vi "art联动采集V4.3.vi"() -> ()   [LabVIEW 2016]
uses:
  <vilib>/Instr/_visa.llb/VISA Configure Serial Port (Instr).vi
  <vilib>/Utility/file.llb/Write Delimited Spreadsheet (DBL).vi
panel:
  in  "定位模式":bool
  in  "X终点":dbl
  in  "Y终点":dbl
  in  "高级设置":bool
  in  "Y轴回零速度":dbl=15000.0
  in  "X轴回零速度":dbl=15000.0
  in  "细分设置":dbl=8.0
  in  "等待时间":u32=40
  in  "文件保存":path=path "C:/Users/H301/Desktop/art采集实验数据" caption="保存路径"
  out "行用时（s）":dbl
  out "time（行）":u32
  out "hDevice out":i32=253955776
  out "error out":errorcluster caption="错误输出"
  in  "退出扫描(Esc)":bool
  in  "N_Length":i32=16384
  out "M_Length":i32
  out "hDevice":i32=241832032
  out "pulDDR2Length":u32=256
  out "总用时（s）":dbl
  out "毫秒计时值":u32=3586537
  out "数组":dbl[][](array[numeric])=[[58819.77200735986, 88200.32943600747]]
  out "强度图":dbl[][](graph)=[[58819.77200735986, 88200.32943600747]]
  out "judge":dbl
  out "Xloop":dbl
  out "幅频谱":dbl[](graph)
  out "时域谱":dbl[](graph)
  out "错误输出":errorcluster
  in  "启动":bool
  in  "开始扫描":bool
  in  "X归零":bool
  in  "Y归零":bool
  in  "Y起点":dbl
  in  "Y轴速度":dbl=9000.0
  in  "X轴速度":dbl=9000.0
  out "电机状态":bool
  in  "电机端口":refnum<visa-resource-name>="COM6"
  out "Yloop":dbl=1.0
  out "X扫描范围":dbl=150.0
  out "Y扫描范围":dbl=75.0
  out "Y序":i32
  in  "X起点":dbl
  out "Y(mm)":dbl
  out "x+y 2":dbl=3.0
  in  "Y步进":dbl=1.0
  in  "精度":dbl=0.001
  in  "电机急停":bool
  out "X（mm）":dbl
  out "x+y":dbl=1.0
  in  "X步进":dbl=1.0
  # "实时坐标"
  # "时域谱"
  # "频域谱"
  # "扫描参数"
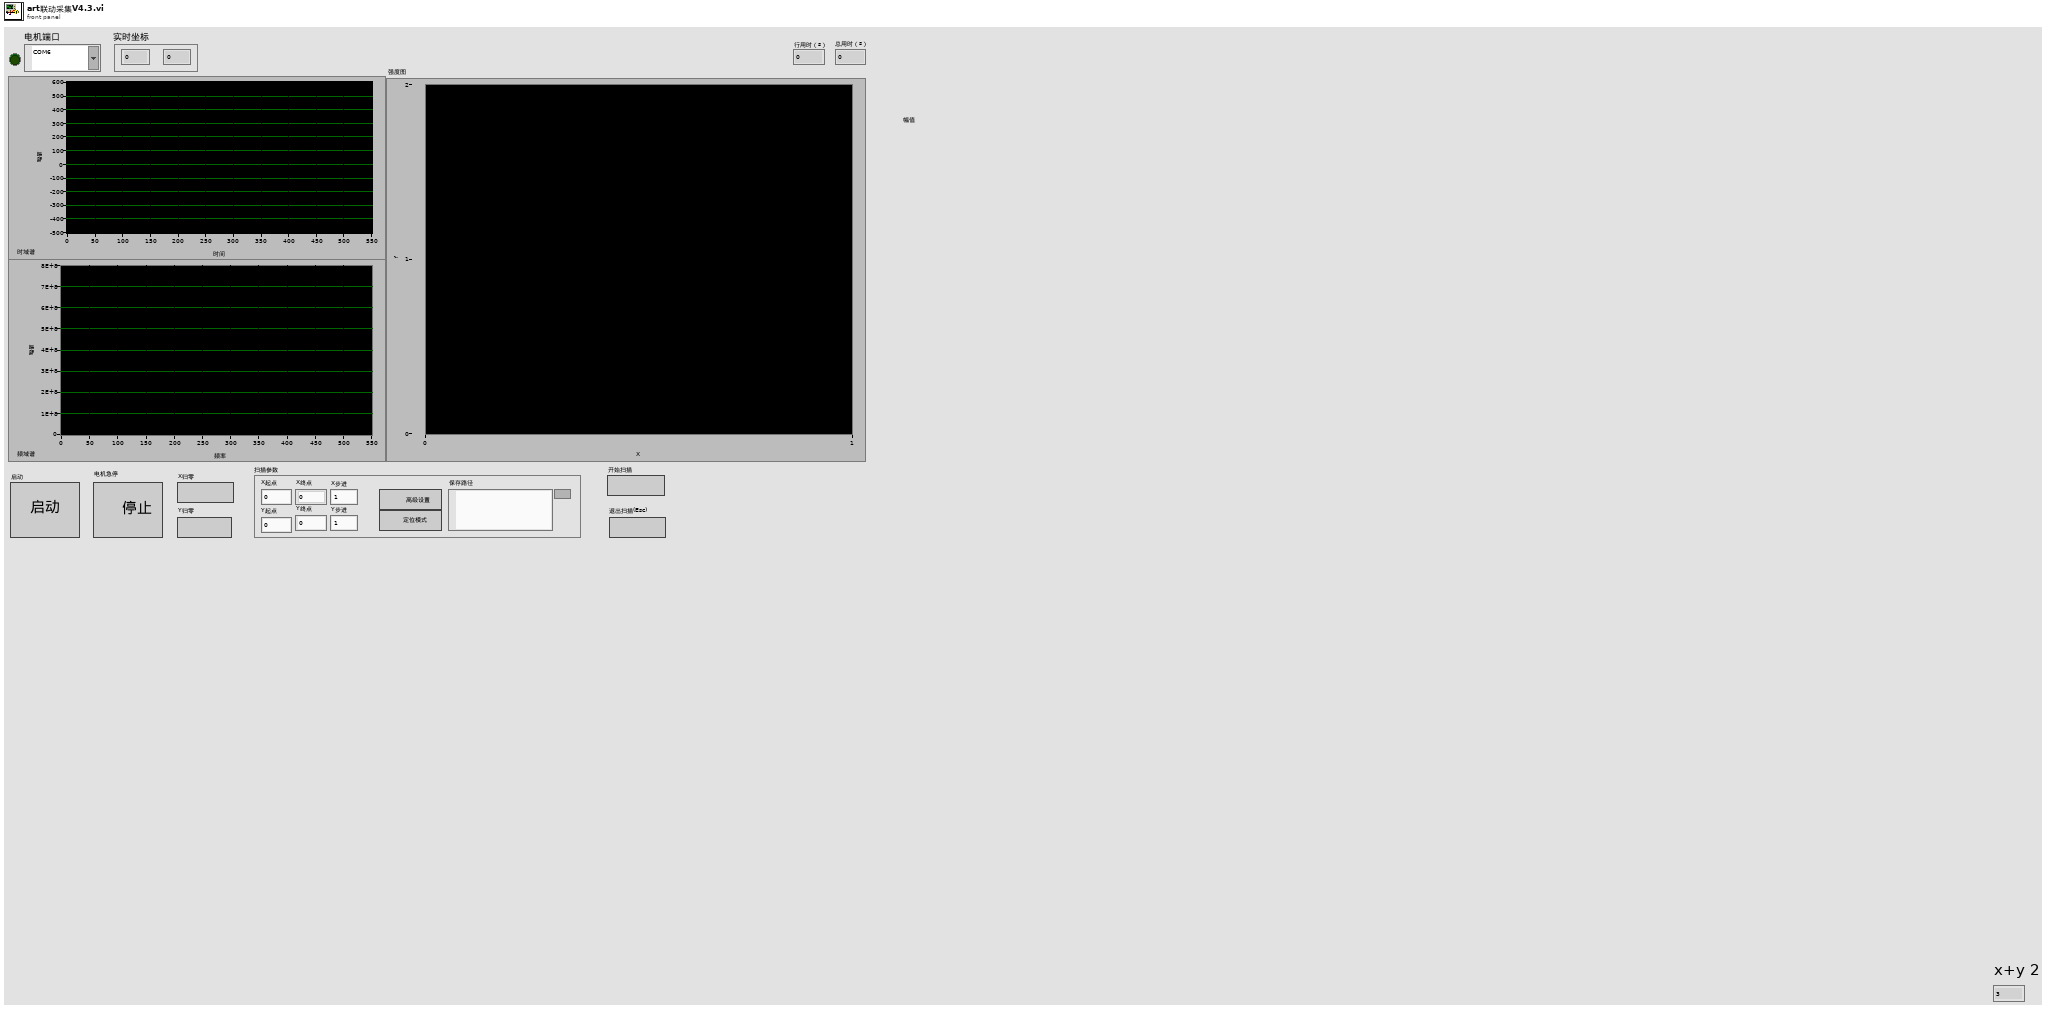
[diagram p1: front panel]
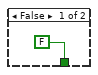
[diagram p2: hidden frame]
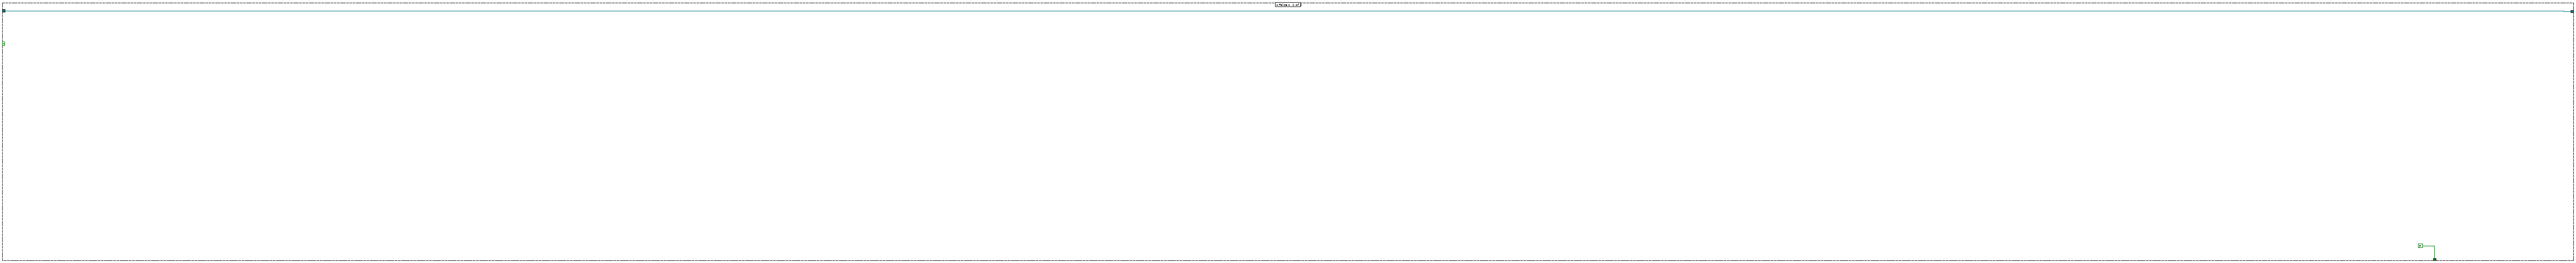
[diagram p3: hidden frame]
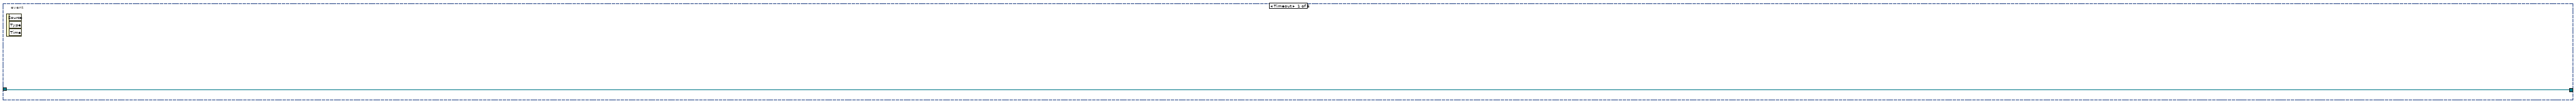
[diagram p4: hidden frame]
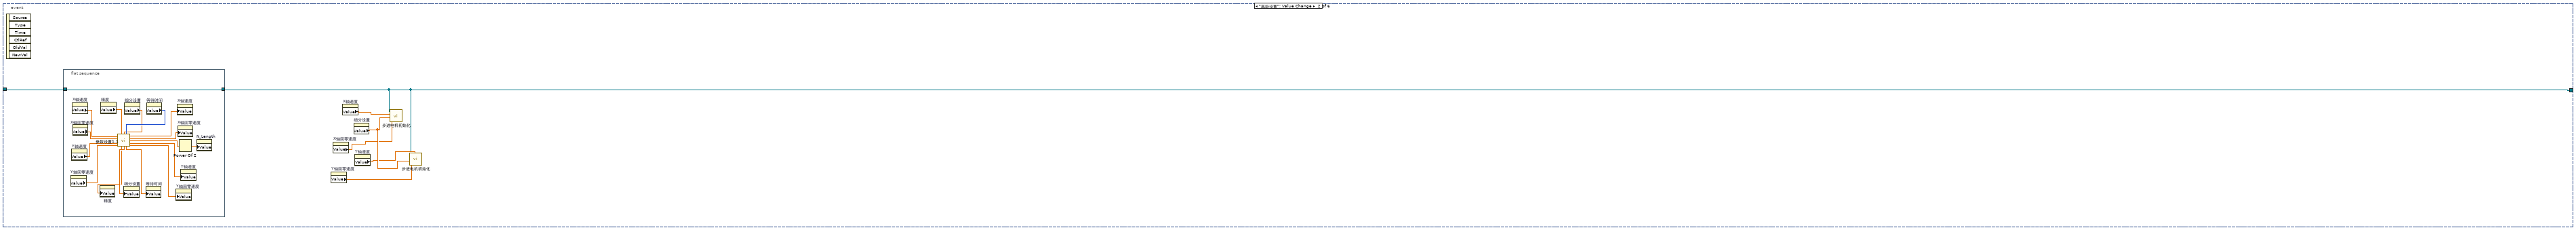
[diagram p5: hidden frame]
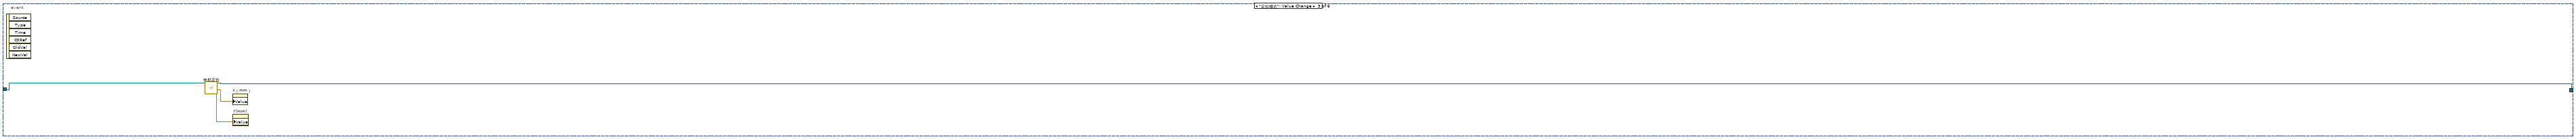
[diagram p6: hidden frame]
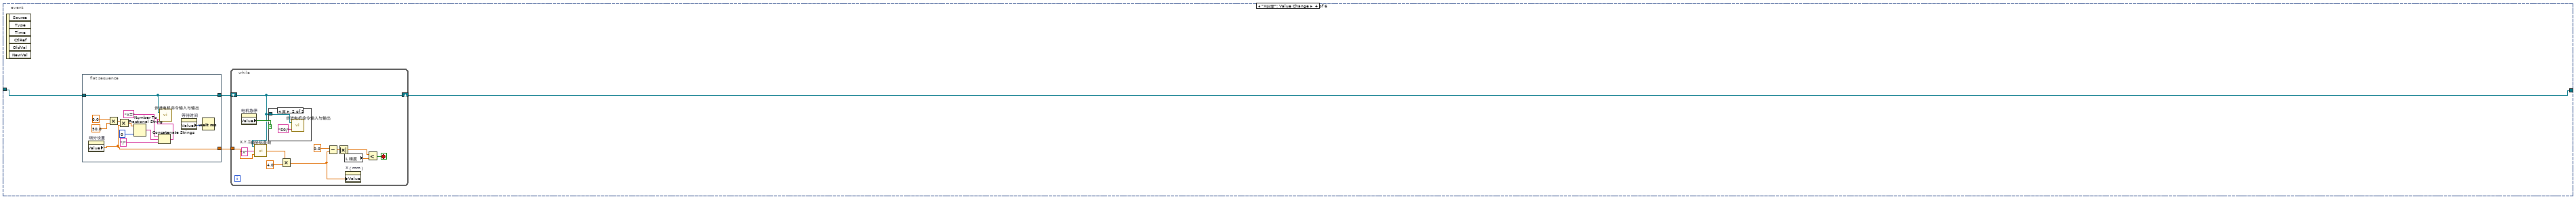
[diagram p7: hidden frame]
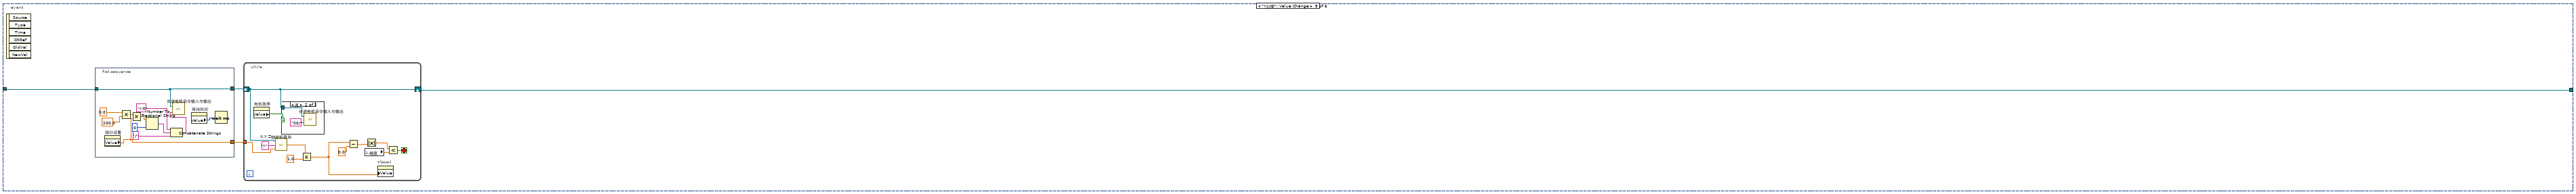
[diagram p9: hidden frame]
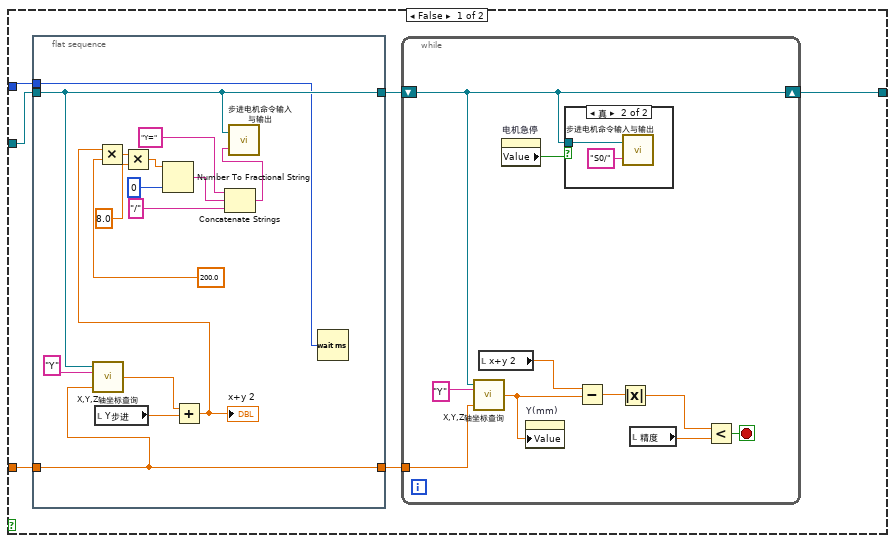
[diagram p14: hidden frame]
diagram:
  n1 = while {
    stop <- w3 stop-if-true
    n2 = case shown="真" "启动" {
      tunnel: [FALSE ("ESC") w11] -> w3
      frame False {
      }
      frame True {
        w25 = 0  # OutClockSource
        w26 = 0  # bClockSourceDir
        w28 = 10000000  # Frequency
        w29 = 0  # ClockSource
        w30 = 0  # TrigLevelVolt
        w18 = 1
        w31 = 0  # TriggerDir
        w32 = 0  # TriggerSource
        w33 = 0  # ATRTriggerChannel
        w34 = 0  # TriggerMode
        w19 = 0  # M_Length
        w35 = 1  # CouplingType
        w36 = 0  # DeviceLgcID
        w46 = u16 0 items=["无", "XON/XOFF", "RTS/CTS", "XON/XOFF & RTS/CTS", "DTR/DSR", "XON/XOFF & DTR/DSR"] ("flow control (0:none)")
        w47 = u16 10 items=["1.0"=10, "1.5"=15, "2.0"=20] ("stop bits (10: 1 bit)")
        # "3"
        # "2"
        # "1"
        n3 = call-poly "VISA Configure Serial Port"("VISA resource name"="电机端口", "baud rate (9600)"=u32 9600, "data bits (8)"=u16 8, "parity (0:none)"=enum16{"None", "Odd", "Even", "Mark", "Space"}."None", "stop bits (10: 1 bit)"=w47, "flow control (0:none)"=w46) -> ("VISA resource name out"=w38:refnum<visa-resource-name>, "error out"=→"error out":errorcluster)  [unwired: 1 in, 7 out]
        n4 = Build Array "InputRange"(w18, w18, w18, w18) -> (w17:i32[])
        n5 = dll-call lib="PTH2aabs CUsersH301Desktopart闭环扫描程序采集卡控制INFamd64PCI8502_32.dll" fn="PCI8502_CreateDevice" label="CreateDevice"("DeviceLgcID"=w36) -> (w23:i32)  [unwired: 4 in, 2 out]
        n6 = property on="细分设置" class="DigNum (严格)"() -> ("Value"=w10:dbl)  [unwired: 2 in, 2 out]
        n7 = Build Array (concatenate) "InitDeviceAD"(w28, w17, w35, w19, "N_Length", w34, w33, w32, w31, w30, w29, w26, w25) -> (w27:i32[])
        n8 = call "步进电机初始化.vi"("回零速度"="X轴回零速度", "细分设置"=w10, "X轴速度"="X轴速度", "串口通信端口"=w38) -> ()  [unwired: 2 in, 1 out]
        n9 = dll-call lib="PTH2aabs CUsersH301Desktopart闭环扫描程序采集卡控制INFamd64PCI8502_32.dll" fn="PCI8502_GetDDR2Length" label="GetDDR2Length"("hDevice"=w23, "pulDDR2Length"=u32 0) -> ("hDevice"=w22:i32, "pulDDR2Length"=→"pulDDR2Length":u32)  [unwired: 4 in, 2 out]
        n10 = call "步进电机初始化.vi"("Y轴速度"="Y轴速度", "回零速度"="Y轴回零速度", "细分设置"=w10, "串口通信端口"=w38) -> ()  [unwired: 2 in, 1 out]
        n11 = call "步进电机命令输入与输出.vi"("输入字符串"="?R/", "串口通信端口"=w38) -> ("返回字符串"=w43:string)
        n12 = dll-call lib="PTH2aabs CUsersH301Desktopart闭环扫描程序采集卡控制INFamd64PCI8502_32.dll" fn="PCI8502_InitDeviceAD" label="InitDeviceAD"("hDevice"=w22, "pADPara"=w27) -> ("hDevice"=→"hDevice":i32)  [unwired: 5 in, 2 out]
        n13 = String Subset(string=w43, offset (0)=0 ("偏移量(0)"), length (rest)=2 ("长度（剩余）")) -> (substring=w40:string)
        n14 = Equal?(x=w40, y="OK") -> (x = y?=w37:bool)
        "电机状态" <- w37
        n15 = case shown="真" w37 {
          tunnel: w38 -> [w53 w56]
          tunnel: [w53 w54] -> w12
          tunnel: [FALSE ("ESC") w55] -> w11
          frame False {
          }
          frame True {
            n16 = while {
              tunnel: ["退出扫描(Esc)"] -> w55
              shift-right: [w57] -> w54
              shift-left: w56 -> [w62]
              stop <- "退出扫描(Esc)" stop-if-true
              n17 = property on="高级设置" class="Bool"("Visible"=TRUE ("可见")) -> ()  [unwired: 2 in, 2 out]
              n18 = property on="定位模式" class="Bool"("Visible"=TRUE ("可见")) -> ()  [unwired: 2 in, 2 out]
              n19 = event shown="[5] \"开始扫描\": 值改变" {
                selector: _ -> [_ _ _ _ _ _]
                dyn-events: _ -> [_ _ _ _ _ _]
                timeout: 1 -> [_ _ _ _ _ _]
                tunnel: w62 -> [w63 w70 w91 w95 w125 w176]
                tunnel: [w63 w64 w90 w93 w123 w170] -> w57
                event Timeout {
                  n20 = event-data() -> ()  [unwired: 1 in, 3 out]
                }
                event "高级设置": Value Change {
                  n21 = event-data() -> ()  [unwired: 1 in, 6 out]
                  n22 = flat-sequence {
                    tunnel: w70 -> [w73]
                    tunnel: [w73] -> w64
                    frame #0 {
                      n23 = property on="Y轴回零速度" class="DigNum (严格)"() -> ("Value"=w77:dbl)  [unwired: 2 in, 2 out]
                      n24 = property on="Y轴速度" class="DigNum (严格)"() -> ("Value"=w76:dbl)  [unwired: 2 in, 2 out]
                      n25 = property on="X轴速度" class="DigNum (严格)"() -> ("Value"=w74:dbl)  [unwired: 2 in, 2 out]
                      n26 = property on="X轴回零速度" class="DigNum (严格)"() -> ("Value"=w75:dbl)  [unwired: 2 in, 2 out]
                      n27 = property on="精度" class="DigNum (严格)"() -> ("Value"=w81:dbl)  [unwired: 2 in, 2 out]
                      n28 = property on="细分设置" class="DigNum (严格)"() -> ("Value"=w82:dbl)  [unwired: 2 in, 2 out]
                      n29 = property on="等待时间" class="DigNum (严格)"() -> ("Value"=w83:u32)  [unwired: 2 in, 2 out]
                      n30 = call "参数设置1.1.vi"("X轴速度"=w74, "精度"=w81, "细分设置"=w82, "等待时间"=w83, "X轴回零速度"=w75, "Y轴速度"=w76, "Y轴回零速度"=w77) -> ("X轴速度"=w84:dbl, "X轴回零速度"=w85:dbl, "采样阶"=w71:dbl, "Y轴速度"=w86:dbl, "精度"=w78:dbl, "细分设置"=w79:dbl, "等待时间"=w80:dbl, "Y轴回零速度"=w87:dbl)  [unwired: 1 in]
                      n31 = property on="精度" class="DigNum (严格)"("Value"=w78) -> ()  [unwired: 2 in, 2 out]
                      n32 = property on="细分设置" class="DigNum (严格)"("Value"=w79) -> ()  [unwired: 2 in, 2 out]
                      n33 = property on="等待时间" class="DigNum (严格)"("Value"=w80) -> ()  [unwired: 2 in, 2 out]
                      n34 = property on="Y轴回零速度" class="DigNum (严格)"("Value"=w87) -> ()  [unwired: 2 in, 2 out]
                      n35 = property on="X轴速度" class="DigNum (严格)"("Value"=w84) -> ()  [unwired: 2 in, 2 out]
                      n36 = property on="X轴回零速度" class="DigNum (严格)"("Value"=w85) -> ()  [unwired: 2 in, 2 out]
                      n37 = Power Of 2(x=w71) -> (2^x=w72:dbl)
                      n38 = property on="Y轴速度" class="DigNum (严格)"("Value"=w86) -> ()  [unwired: 2 in, 2 out]
                      n39 = property on="N_Length" class="DigNum (严格)"("Value"=w72) -> ()  [unwired: 2 in, 2 out]
                    }
                  }
                  n40 = property on="Y轴回零速度" class="DigNum (严格)"() -> ("Value"=w66:dbl)  [unwired: 2 in, 2 out]
                  n41 = property on="X轴回零速度" class="DigNum (严格)"() -> ("Value"=w67:dbl)  [unwired: 2 in, 2 out]
                  n42 = property on="X轴速度" class="DigNum (严格)"() -> ("Value"=w68:dbl)  [unwired: 2 in, 2 out]
                  n43 = property on="细分设置" class="DigNum (严格)"() -> ("Value"=w69:dbl)  [unwired: 2 in, 2 out]
                  n44 = property on="Y轴速度" class="DigNum (严格)"() -> ("Value"=w65:dbl)  [unwired: 2 in, 2 out]
                  n45 = call "步进电机初始化.vi"("回零速度"=w67, "细分设置"=w69, "X轴速度"=w68, "串口通信端口"=w64) -> ()  [unwired: 2 in, 1 out]
                  n46 = call "步进电机初始化.vi"("Y轴速度"=w65, "回零速度"=w66, "细分设置"=w69, "串口通信端口"=w64) -> ()  [unwired: 2 in, 1 out]
                }
                event "定位模式": Value Change {
                  n47 = event-data() -> ()  [unwired: 1 in, 6 out]
                  n48 = call "电机定位.vi"("VISA I"=w91) -> ("Y"=w88:dbl, "X"=w89:dbl, "VISA O"=w90:refnum<visa-resource-name>)  [unwired: 8 in]
                  n49 = property on="X（mm）" class="DigNum (严格)"("Value"=w89) -> ()  [unwired: 2 in, 2 out]
                  n50 = property on="Y(mm)" class="DigNum (严格)"("Value"=w88) -> ()  [unwired: 2 in, 2 out]
                }
                event "X归零": Value Change {
                  n51 = event-data() -> ()  [unwired: 1 in, 6 out]
                  n52 = flat-sequence {
                    tunnel: w95 -> [w99]
                    tunnel: [w99] -> w94
                    tunnel: [w96] -> w92
                    frame #0 {
                      n53 = property on="细分设置" class="DigNum (严格)"() -> ("Value"=w96:dbl)  [unwired: 2 in, 2 out]
                      n54 = Multiply(x=0.0, y=50.0) -> (x*y=w102:dbl)
                      n55 = Multiply(x=w102, y=w96) -> (x*y=w107:dbl)
                      n56 = Number To Fractional String(number=w107, precision (6)=i16 0 ("精度(6)")) -> (F-format string=w105:string)  [unwired: 2 out]
                      n57 = Concatenate Strings("X=" ("字符串"), w105, "/" ("字符串")) -> (w100:string)
                      n58 = call "步进电机命令输入与输出.vi"("输入字符串"=w100, "串口通信端口"=w99) -> ()  [unwired: 1 out]
                      n59 = property on="等待时间" class="DigNum (严格)"() -> ("Value"=w97:u32)  [unwired: 2 in, 2 out]
                      n60 = Wait (ms)(milliseconds to wait=w97) -> ()  [unwired: 1 out]
                    }
                  }
                  n61 = while {
                    tunnel: w92 -> [w108]
                    shift-right: [w109] -> w93
                    shift-left: w94 -> [w109]
                    stop <- w115 stop-if-true
                    n62 = property on="电机急停" class="Bool (严格)"() -> ("Value"=w116:bool)  [unwired: 2 in, 2 out]
                    n63 = call "X,Y,Z轴坐标查询.vi"("细分设置"=w108, "查询坐标轴"="X", "串口通信端口"=w109) -> ("坐标(mm)"=w117:dbl)
                    n64 = case shown="真" w116 {
                      tunnel: w109 -> [_ w120]
                      frame False {
                      }
                      frame True {
                        n65 = call "步进电机命令输入与输出.vi"("输入字符串"="S0/", "串口通信端口"=w120) -> ()  [unwired: 1 out]
                      }
                    }
                    n66 = Multiply(x=w117, y=4.0 ("x")) -> (x*y=w113:dbl)
                    n67 = Subtract(x=0.0, y=w113) -> (x-y=w112:dbl)
                    n68 = Absolute Value(x=w112) -> (abs(x)=w111:dbl)
                    n69 = local read "精度"() -> (w114:dbl)
                    n70 = property on="X（mm）" class="DigNum (严格)"("Value"=w113) -> ()  [unwired: 2 in, 2 out]
                    n71 = Less?(x=w111, y=w114) -> (x < y?=w115:bool)
                  }
                }
                event "Y归零": Value Change {
                  n72 = event-data() -> ()  [unwired: 1 in, 6 out]
                  n73 = flat-sequence {
                    tunnel: w125 -> [w129]
                    tunnel: [w129] -> w124
                    tunnel: [w126] -> w122
                    frame #0 {
                      n74 = property on="细分设置" class="DigNum (严格)"() -> ("Value"=w126:dbl)  [unwired: 2 in, 2 out]
                      n75 = Multiply(x=0.0, y=200.0) -> (x*y=w132:dbl)
                      n76 = Multiply(x=w132, y=w126) -> (x*y=w137:dbl)
                      n77 = Number To Fractional String(number=w137, precision (6)=i16 0 ("精度(6)")) -> (F-format string=w135:string)  [unwired: 2 out]
                      n78 = Concatenate Strings("Y=" ("字符串"), w135, "/" ("字符串")) -> (w130:string)
                      n79 = call "步进电机命令输入与输出.vi"("输入字符串"=w130, "串口通信端口"=w129) -> ()  [unwired: 1 out]
                      n80 = property on="等待时间" class="DigNum (严格)"() -> ("Value"=w127:u32)  [unwired: 2 in, 2 out]
                      n81 = Wait (ms)(milliseconds to wait=w127) -> ()  [unwired: 1 out]
                    }
                  }
                  n82 = while {
                    tunnel: w122 -> [w138]
                    shift-right: [w139] -> w123
                    shift-left: w124 -> [w139]
                    stop <- w145 stop-if-true
                    n83 = property on="电机急停" class="Bool (严格)"() -> ("Value"=w146:bool)  [unwired: 2 in, 2 out]
                    n84 = call "X,Y,Z轴坐标查询.vi"("细分设置"=w138, "查询坐标轴"="Y", "串口通信端口"=w139) -> ("坐标(mm)"=w147:dbl)
                    n85 = case shown="真" w146 {
                      tunnel: w139 -> [_ w150]
                      frame False {
                      }
                      frame True {
                        n86 = call "步进电机命令输入与输出.vi"("输入字符串"="S0/", "串口通信端口"=w150) -> ()  [unwired: 1 out]
                      }
                    }
                    n87 = Multiply(x=w147, y=1.0 ("x")) -> (x*y=w143:dbl)
                    n88 = Subtract(x=w143, y=0.0 ("x")) -> (x-y=w141:dbl)
                    n89 = local read "精度"() -> (w144:dbl)
                    n90 = Absolute Value(x=w141) -> (abs(x)=w140:dbl)
                    n91 = property on="Y(mm)" class="DigNum (严格)"("Value"=w143) -> ()  [unwired: 2 in, 2 out]
                    n92 = Less?(x=w140, y=w144) -> (x < y?=w145:bool)
                  }
                }
                event "开始扫描": Value Change {
                  n93 = event-data() -> ()  [unwired: 1 in, 6 out]
                  n94 = flat-sequence {
                    tunnel: w176 -> [w193]
                    tunnel: [w193] -> w166
                    frame #0 {
                      # "如果强度图那里出了错，就把这里的行列互换"
                      n95 = local read "Xloop"() -> (w188:dbl)
                      n96 = local read "Yloop"() -> (w187:dbl)
                      n97 = Multiply(x="Y起点", y=200.0) -> (x*y=w196:dbl)
                      n98 = Tick Count (ms)() -> (millisecond timer value=→"毫秒计时值":u32)
                      n99 = Multiply(x=w196, y="细分设置") -> (x*y=w201:dbl)
                      n100 = Initialize Array(0.0 ("元素"), w188, w187) -> (→"强度图":dbl[][])
                      n101 = Number To Fractional String(number=w201, precision (6)=i16 0 ("精度(6)")) -> (F-format string=w199:string)  [unwired: 2 out]
                      n102 = Concatenate Strings("Y=" ("字符串"), w199, "/" ("字符串")) -> (w194:string)
                      n103 = call "步进电机命令输入与输出.vi"("输入字符串"=w194, "串口通信端口"=w193) -> ()  [unwired: 1 out]
                      n104 = property on="等待时间" class="DigNum (严格)"() -> ("Value"=w185:u32)  [unwired: 2 in, 2 out]
                      n105 = Wait (ms)(milliseconds to wait=w185) -> ()  [unwired: 1 out]
                    }
                  }
                  n106 = local read "X起点"() -> (w162:dbl)
                  n107 = Subtract(x="X终点", y=w162) -> (x-y=w161:dbl)
                  "X扫描范围" <- w161
                  n108 = local read "X步进"() -> (w169:dbl)
                  n109 = Divide(x=w161, y=w169) -> (x/y=w167:dbl)
                  n110 = Increment(x=w167) -> (x+1=→"Xloop":dbl)
                  n111 = while {
                    shift-right: [w202] -> w152
                    shift-left: w166 -> [w202]
                    stop <- w207 stop-if-true
                    n112 = call "X,Y,Z轴坐标查询.vi"("细分设置"=8.0, "查询坐标轴"="Y", "串口通信端口"=w202) -> ("坐标(mm)"=w209:dbl)
                    n113 = property on="Y起点" class="DigNum (严格)"() -> ("Value"=w211:dbl)  [unwired: 2 in, 2 out]
                    n114 = property on="电机急停" class="Bool (严格)"() -> ("Value"=w208:bool)  [unwired: 2 in, 2 out]
                    n115 = Multiply(x=w209, y=1.0 ("x")) -> (x*y=w205:dbl)
                    n116 = Subtract(x=w211, y=w205) -> (x-y=w204:dbl)
                    n117 = case shown="真" w208 {
                      tunnel: w202 -> [_ w214]
                      frame False {
                      }
                      frame True {
                        n118 = call "步进电机命令输入与输出.vi"("输入字符串"="S0/", "串口通信端口"=w214) -> ()  [unwired: 1 out]
                      }
                    }
                    n119 = Absolute Value(x=w204) -> (abs(x)=w203:dbl)
                    n120 = local read "精度"() -> (w206:dbl)
                    n121 = property on="Y(mm)" class="DigNum (严格)"("Value"=w205) -> ()  [unwired: 2 in, 2 out]
                    n122 = Less?(x=w203, y=w206) -> (x < y?=w207:bool)
                  }
                  n123 = local read "Y起点"() -> (w164:dbl)
                  n124 = local read "Y步进"() -> (w175:dbl)
                  n125 = Subtract(x="Y终点", y=w164) -> (x-y=w160:dbl)
                  "Y扫描范围" <- w160
                  n126 = Divide(x=w160, y=w175) -> (x/y=w174:dbl)
                  n127 = Increment(x=w174) -> (x+1=w173:dbl)
                  "Yloop" <- w173
                  n128 = Build Path(base path="文件保存", name or relative path="频域谱" ("名称或相对路径")) -> (appended path=w157:path)
                  n129 = Create Folder(path (use dialog)=w157) -> (created path=w153:path)  [unwired: 2 in, 2 out]
                  n130 = Build Path(base path="文件保存", name or relative path="时域谱" ("名称或相对路径")) -> (appended path=w159:path)
                  n131 = Create Folder(path (use dialog)=w159) -> (created path=w154:path)  [unwired: 2 in, 2 out]
                  n132 = for {
                    N: w173 -> [_]
                    shift-right: [w238] -> w172
                    shift-left: w152 -> [w218]
                    tunnel: [w220] -> w171 mode=indexing
                    tunnel: w154 -> [w224]
                    tunnel: w153 -> [w223]
                    i -> [w239]
                    # "实时成像出问题调这里"
                    n133 = flat-sequence {
                      tunnel: w218 -> [w296]
                      tunnel: [w296] -> w237
                      tunnel: [w292] -> w228
                      frame #0 {
                        n134 = property on="细分设置" class="DigNum (严格)"() -> ("Value"=w292:dbl)  [unwired: 2 in, 2 out]
                        n135 = Multiply(x="X起点", y=50.0) -> (x*y=w299:dbl)
                        n136 = Multiply(x=w299, y=w292) -> (x*y=w304:dbl)
                        n137 = Number To Fractional String(number=w304, precision (6)=i16 0 ("精度(6)")) -> (F-format string=w302:string)  [unwired: 2 out]
                        n138 = Concatenate Strings("X=" ("字符串"), w302, "/" ("字符串")) -> (w297:string)
                        n139 = call "步进电机命令输入与输出.vi"("输入字符串"=w297, "串口通信端口"=w296) -> ()  [unwired: 1 out]
                        n140 = Tick Count (ms)() -> (millisecond timer value=→"time（行）":u32)
                        n141 = Wait (ms)(milliseconds to wait="等待时间") -> ()  [unwired: 1 out]
                      }
                    }
                    n142 = while {
                      tunnel: w228 -> [w306]
                      shift-right: [w305] -> w216
                      shift-left: w237 -> [w305]
                      stop <- w311 stop-if-true
                      n143 = property on="电机急停" class="Bool (严格)"() -> ("Value"=w312:bool)  [unwired: 2 in, 2 out]
                      n144 = case shown="真" w312 {
                        tunnel: w305 -> [_ w317]
                        frame False {
                        }
                        frame True {
                          n145 = call "步进电机命令输入与输出.vi"("输入字符串"="S0/", "串口通信端口"=w317) -> ()  [unwired: 1 out]
                        }
                      }
                      n146 = call "X,Y,Z轴坐标查询.vi"("细分设置"=w306, "查询坐标轴"="X", "串口通信端口"=w305) -> ("坐标(mm)"=w313:dbl)
                      n147 = Multiply(x=w313, y=4.0 ("x")) -> (x*y=w309:dbl)
                      n148 = property on="X起点" class="DigNum (严格)"() -> ("Value"=w315:dbl)  [unwired: 2 in, 2 out]
                      n149 = Subtract(x=w315, y=w309) -> (x-y=w308:dbl)
                      n150 = Absolute Value(x=w308) -> (abs(x)=w307:dbl)
                      n151 = local read "精度"() -> (w310:dbl)
                      n152 = property on="X（mm）" class="DigNum (严格)"("Value"=w309) -> ()  [unwired: 2 in, 2 out]
                      n153 = Less?(x=w307, y=w310) -> (x < y?=w311:bool)
                    }
                    n154 = local read "Xloop"() -> (w229:dbl)
                    n155 = for {
                      N: w229 -> [_]
                      shift-right: [w390] -> w217
                      shift-left: w216 -> [w385]
                      tunnel: [w389] -> w236 mode=indexing
                      tunnel: [w388] -> w235 mode=indexing
                      tunnel: [w387] -> w220 mode=indexing
                      i -> [w386]
                      n156 = flat-sequence {
                        tunnel: w385 -> [w395]
                        tunnel: [w394] -> w391
                        tunnel: w386 -> [w392]
                        tunnel: [w453] -> w390
                        tunnel: w391 -> [w453]
                        tunnel: [w452] -> w389
                        tunnel: [w451] -> w388
                        tunnel: [w449] -> w387
                        frame #0 {
                          n157 = Equal To 0?(x=w392) -> (x = 0?=w393:bool)
                          n158 = case shown="假" w393 {
                            tunnel: w395 -> [w398 w433]
                            tunnel: [w397 w433] -> w394
                            frame False {
                              n159 = flat-sequence {
                                tunnel: w398 -> [w408]
                                tunnel: [w408] -> w399
                                tunnel: [w400] -> w396
                                frame #0 {
                                n160 = local read "X步进"() -> (w402:dbl)
                                n161 = Multiply(x=w402, y=1.0 ("x")) -> (x*y=w407:dbl)
                                n162 = property on="等待时间" class="DigNum (严格)"() -> ("Value"=w401:u32)  [unwired: 2 in, 2 out]
                                n163 = property on="细分设置" class="DigNum (严格)"() -> ("Value"=w400:dbl)  [unwired: 2 in, 2 out]
                                n164 = call "X,Y,Z轴坐标查询.vi"("细分设置"=w400, "查询坐标轴"="X", "串口通信端口"=w408) -> ("坐标(mm)"=w404:dbl)
                                n165 = Multiply(x=4.0, y=w404) -> (x*y=w403:dbl)
                                n166 = Add(x=w403, y=w407) -> (x+y=w410:dbl)
                                "x+y" <- w410
                                n167 = Multiply(x=w410, y=50.0) -> (x*y=w413:dbl)
                                n168 = Multiply(x=w413, y=w400) -> (x*y=w418:dbl)
                                n169 = Number To Fractional String(number=w418, precision (6)=i16 0 ("精度(6)")) -> (F-format string=w416:string)  [unwired: 2 out]
                                n170 = Concatenate Strings("X=" ("字符串"), w416, "/" ("字符串")) -> (w411:string)
                                n171 = call "步进电机命令输入与输出.vi"("输入字符串"=w411, "串口通信端口"=w408) -> ()  [unwired: 1 out]
                                n172 = Wait (ms)(milliseconds to wait=w401) -> ()  [unwired: 1 out]
                                }
                              }
                              n173 = while {
                                tunnel: w396 -> [w419]
                                shift-right: [w428] -> w397
                                shift-left: w399 -> [w428]
                                stop <- w427 stop-if-true
                                n174 = property on="电机急停" class="Bool (严格)"() -> ("Value"=w425:bool)  [unwired: 2 in, 2 out]
                                n175 = local read "x+y"() -> (w429:dbl)
                                n176 = case shown="真" w425 {
                                tunnel: w428 -> [_ w431]
                                frame False {
                                }
                                frame True {
                                n177 = call "步进电机命令输入与输出.vi"("输入字符串"="S0/", "串口通信端口"=w431) -> ()  [unwired: 1 out]
                                }
                                }
                                n178 = call "X,Y,Z轴坐标查询.vi"("细分设置"=w419, "查询坐标轴"="X", "串口通信端口"=w428) -> ("坐标(mm)"=w423:dbl)
                                n179 = Multiply(x=4.0, y=w423) -> (x*y=w422:dbl)
                                n180 = Subtract(x=w429, y=w422) -> (x-y=w421:dbl)
                                n181 = property on="X（mm）" class="DigNum (严格)"("Value"=w422) -> ()  [unwired: 2 in, 2 out]
                                n182 = Absolute Value(x=w421) -> (abs(x)=w420:dbl)
                                n183 = local read "精度"() -> (w424:dbl)
                                n184 = Less?(x=w420, y=w424) -> (x < y?=w427:bool)
                              }
                            }
                            frame True {
                            }
                          }
                        }
                        frame #1 {
                          n185 = local read "pulDDR2Length"() -> (w448:u32)
                          n186 = local read "hDevice"() -> (w447:i32)
                          n187 = local read "M_Length"() -> (w445:i32)
                          n188 = property on="N_Length" class="DigNum (严格)"() -> ("Value"=w434:i32)  [unwired: 2 in, 2 out]
                          n189 = Subtract(x=w434, y=w445) -> (x-y=w443:i32)
                          n190 = Multiply(x=w443, y=0.25) -> (x*y=w436:dbl)
                          n191 = Multiply(x=w436, y=0.442) -> (x*y=w438:dbl)
                          n192 = Multiply(x=w436, y=0.058) -> (x*y=w440:dbl)
                          n193 = Round Toward -Infinity(1:w438) -> (0:w435:dbl)
                          n194 = Round Toward -Infinity(1:w440) -> (0:w439:dbl)
                          n195 = call "AD（V3.2）.vi"("N-length"=w434, "M-length"=w445, "hDevice"=w447, "pulDDR2Length"=w448) -> ("幅频谱"=w451:dbl[], "时域谱"=w452:dbl[], "hDevice out"=→"hDevice out":i32)  [unwired: 5 in]
                          "时域谱" <- w452
                          "幅频谱" <- w451
                          n196 = Increment(x=w435) -> (x+1=w442:dbl)
                          n197 = Array Subset(array=w451, index=w439, length=w442) -> (w450:dbl[])
                          n198 = Array Max & Min(array=w450) -> (max value=w449:dbl)  [unwired: 3 out]
                        }
                      }
                    }
                    n199 = flat-sequence {
                      tunnel: w235 -> [w273]
                      tunnel: w236 -> [w281]
                      tunnel: w217 -> [w290]
                      tunnel: [w290] -> w231
                      tunnel: w224 -> [w268]
                      tunnel: w223 -> [w267]
                      frame #0 {
                        n200 = local read "time（行）"() -> (w289:u32)
                        n201 = Tick Count (ms)() -> (millisecond timer value=w285:u32)
                        n202 = Subtract(x=w285, y=w289) -> (x-y=w288:u32)
                        n203 = local read "Y序"() -> (w269:i32)
                        n204 = Multiply(x=w288, y=0.001) -> (x*y=→"行用时（s）":dbl)
                        n205 = Increment(x=w269) -> (x+1=w270:i32)
                        n206 = Number To Decimal String(number=w270) -> (decimal integer string=w279:string)  [unwired: 1 in]
                        n207 = Number To Decimal String(number=w270) -> (decimal integer string=w278:string)  [unwired: 1 in]
                        n208 = Concatenate Strings("T" ("字符串"), w279, ".txt" ("字符串")) -> (w282:string)
                        n209 = Concatenate Strings("F" ("字符串"), w278, ".txt" ("字符串")) -> (w276:string)
                        n210 = Build Path(base path=w268, name or relative path=w282) -> (appended path=w284:path)
                        n211 = call-poly <vilib>:"Write Delimited Spreadsheet.vi"("file path (dialog if empty)"=w284, "2D data"=w281, "transpose? (no:F)"=FALSE) -> ()  [unwired: 11 in, 2 out]
                        n212 = Build Path(base path=w267, name or relative path=w276) -> (appended path=w274:path)
                        n213 = call-poly <vilib>:"Write Delimited Spreadsheet.vi"("file path (dialog if empty)"=w274, "2D data"=w273, "transpose? (no:F)"=FALSE) -> ()  [unwired: 11 in, 2 out]
                        "judge" <- 1.0
                      }
                    }
                    n214 = flat-sequence {
                      tunnel: w231 -> [w244]
                      tunnel: [w244] -> w232
                      tunnel: [w242] -> w227
                      frame #0 {
                        n215 = property on="细分设置" class="DigNum (严格)"() -> ("Value"=w242:dbl)  [unwired: 2 in, 2 out]
                        n216 = property on="等待时间" class="DigNum (严格)"() -> ("Value"=w241:u32)  [unwired: 2 in, 2 out]
                        n217 = Multiply(x=0.0, y=50.0) -> (x*y=w247:dbl)
                        n218 = Multiply(x=w247, y=w242) -> (x*y=w252:dbl)
                        n219 = Wait (ms)(milliseconds to wait=w241) -> ()  [unwired: 1 out]
                        n220 = Number To Fractional String(number=w252, precision (6)=i16 0 ("精度(6)")) -> (F-format string=w250:string)  [unwired: 2 out]
                        n221 = Concatenate Strings("X=" ("字符串"), w250, "/" ("字符串")) -> (w245:string)
                        n222 = call "步进电机命令输入与输出.vi"("输入字符串"=w245, "串口通信端口"=w244) -> ()  [unwired: 1 out]
                      }
                    }
                    n223 = while {
                      tunnel: w227 -> [w253]
                      shift-right: [w254] -> w230
                      shift-left: w232 -> [w254]
                      stop <- w260 stop-if-true
                      n224 = property on="电机急停" class="Bool (严格)"() -> ("Value"=w261:bool)  [unwired: 2 in, 2 out]
                      n225 = call "X,Y,Z轴坐标查询.vi"("细分设置"=w253, "查询坐标轴"="X", "串口通信端口"=w254) -> ("坐标(mm)"=w262:dbl)
                      n226 = case shown="真" w261 {
                        tunnel: w254 -> [_ w265]
                        frame False {
                        }
                        frame True {
                          n227 = call "步进电机命令输入与输出.vi"("输入字符串"="S0/", "串口通信端口"=w265) -> ()  [unwired: 1 out]
                        }
                      }
                      n228 = Multiply(x=w262, y=4.0 ("x")) -> (x*y=w258:dbl)
                      n229 = Subtract(x=0.0, y=w258) -> (x-y=w257:dbl)
                      n230 = Absolute Value(x=w257) -> (abs(x)=w256:dbl)
                      n231 = local read "精度"() -> (w259:dbl)
                      n232 = property on="X（mm）" class="DigNum (严格)"("Value"=w258) -> ()  [unwired: 2 in, 2 out]
                      n233 = Less?(x=w256, y=w259) -> (x < y?=w260:bool)
                    }
                    n234 = property on="强度图" class="IntGraph (严格)"() -> ("Value"=w221:dbl[][])  [unwired: 2 in, 2 out]
                    n235 = local read "Yloop"() -> (w233:dbl)
                    n236 = Decrement(x=w233) -> (x-1=w234:dbl)
                    n237 = local read "Y序"() -> (w219:i32)
                    n238 = Replace Array Subset(array=w221, new element=w220, index (col)=w219) -> (w222:dbl[][])  [unwired: 1 in]
                    n239 = property on="强度图" class="IntGraph (严格)"("Value"=w222) -> ()  [unwired: 2 in, 2 out]
                    n240 = Equal?(x=w219, y=w234) -> (x = y?=w240:bool)
                    n241 = Increment(x=w219) -> ()  [unwired: 1 out]
                    n242 = property on="细分设置" class="DigNum (严格)"() -> ("Value"=w225:dbl)  [unwired: 2 in, 2 out]
                    n243 = property on="等待时间" class="DigNum (严格)"() -> ("Value"=w226:u32)  [unwired: 2 in, 2 out]
                    n244 = case shown="真" w240 {
                      tunnel: w230 -> [w324 w356]
                      tunnel: [w322 w357] -> w238
                      tunnel: w226 -> [w320 w354]
                      tunnel: w225 -> [w319 w353]
                      frame False {
                        n245 = flat-sequence {
                          tunnel: w324 -> [w327]
                          tunnel: [w327] -> w323
                          tunnel: [w325] -> w321
                          tunnel: w320 -> [w326]
                          tunnel: w319 -> [w325]
                          frame #0 {
                            n246 = call "X,Y,Z轴坐标查询.vi"("细分设置"=w325, "查询坐标轴"="Y", "串口通信端口"=w327) -> ("坐标(mm)"=w329:dbl)
                            n247 = local read "Y步进"() -> (w328:dbl)
                            n248 = Add(x=w329, y=w328) -> (x+y=w331:dbl)
                            "x+y 2" <- w331
                            n249 = Multiply(x=w331, y=200.0) -> (x*y=w335:dbl)
                            n250 = Multiply(x=w335, y=8.0 ("细分设置")) -> (x*y=w340:dbl)
                            n251 = Number To Fractional String(number=w340, precision (6)=i16 0 ("精度(6)")) -> (F-format string=w338:string)  [unwired: 2 out]
                            n252 = Concatenate Strings("Y=" ("字符串"), w338, "/" ("字符串")) -> (w333:string)
                            n253 = call "步进电机命令输入与输出.vi"("输入字符串"=w333, "串口通信端口"=w327) -> ()  [unwired: 1 out]
                            n254 = Wait (ms)(milliseconds to wait=w326) -> ()  [unwired: 1 out]
                          }
                        }
                        n255 = while {
                          tunnel: w321 -> [w341]
                          shift-right: [w342] -> w322
                          shift-left: w323 -> [w342]
                          stop <- w348 stop-if-true
                          n256 = call "X,Y,Z轴坐标查询.vi"("细分设置"=w341, "查询坐标轴"="Y", "串口通信端口"=w342) -> ("坐标(mm)"=w346:dbl)
                          n257 = local read "x+y 2"() -> (w349:dbl)
                          n258 = property on="电机急停" class="Bool (严格)"() -> ("Value"=w345:bool)  [unwired: 2 in, 2 out]
                          n259 = property on="Y(mm)" class="DigNum (严格)"("Value"=w346) -> ()  [unwired: 2 in, 2 out]
                          n260 = case shown="真" w345 {
                            tunnel: w342 -> [_ w351]
                            frame False {
                            }
                            frame True {
                              n261 = call "步进电机命令输入与输出.vi"("输入字符串"="S0/", "串口通信端口"=w351) -> ()  [unwired: 1 out]
                            }
                          }
                          n262 = Subtract(x=w349, y=w346) -> (x-y=w344:dbl)
                          n263 = Absolute Value(x=w344) -> (abs(x)=w343:dbl)
                          n264 = local read "精度"() -> (w347:dbl)
                          n265 = Less?(x=w343, y=w347) -> (x < y?=w348:bool)
                        }
                      }
                      frame True {
                        n266 = flat-sequence {
                          tunnel: [w361] -> _
                          tunnel: [w361] -> w358
                          tunnel: w356 -> [w361]
                          tunnel: [w359] -> w355
                          tunnel: w354 -> [w360]
                          tunnel: w353 -> [w359]
                          frame #0 {
                            n267 = Multiply(x=0.0, y=200.0) -> (x*y=w365:dbl)
                            n268 = Multiply(x=w365, y=w359) -> (x*y=w370:dbl)
                            n269 = Number To Fractional String(number=w370, precision (6)=i16 0 ("精度(6)")) -> (F-format string=w368:string)  [unwired: 2 out]
                            n270 = Concatenate Strings("Y=" ("字符串"), w368, "/" ("字符串")) -> (w363:string)
                            n271 = call "步进电机命令输入与输出.vi"("输入字符串"=w363, "串口通信端口"=w361) -> ()  [unwired: 1 out]
                            n272 = Wait (ms)(milliseconds to wait=w360) -> ()  [unwired: 1 out]
                          }
                        }
                        n273 = while {
                          tunnel: w355 -> [w371]
                          shift-right: [w372] -> w357
                          shift-left: w358 -> [w372]
                          stop <- w378 stop-if-true
                          n274 = property on="电机急停" class="Bool (严格)"() -> ("Value"=w379:bool)  [unwired: 2 in, 2 out]
                          n275 = call "X,Y,Z轴坐标查询.vi"("细分设置"=w371, "查询坐标轴"="Y", "串口通信端口"=w372) -> ("坐标(mm)"=w380:dbl)
                          n276 = case shown="真" w379 {
                            tunnel: w372 -> [_ w383]
                            frame False {
                            }
                            frame True {
                              n277 = call "步进电机命令输入与输出.vi"("输入字符串"="S0/", "串口通信端口"=w383) -> ()  [unwired: 1 out]
                            }
                          }
                          n278 = Multiply(x=w380, y=1.0 ("x")) -> (x*y=w376:dbl)
                          n279 = Subtract(x=w376, y=0.0 ("x")) -> (x-y=w374:dbl)
                          n280 = local read "精度"() -> (w377:dbl)
                          n281 = Absolute Value(x=w374) -> (abs(x)=w373:dbl)
                          n282 = property on="Y(mm)" class="DigNum (严格)"("Value"=w376) -> ()  [unwired: 2 in, 2 out]
                          n283 = Less?(x=w373, y=w377) -> (x < y?=w378:bool)
                        }
                      }
                    }
                    "Y序" <- w239
                  }
                  n284 = flat-sequence {
                    tunnel: w172 -> [w179]
                    tunnel: w171 -> [w178]
                    tunnel: [w179] -> w170
                    frame #0 {
                      n285 = local read "毫秒计时值"() -> (w183:u32)
                      n286 = Transpose 2D Array(2D array=w178) -> (transposed array=w177:dbl[][])
                      n287 = Tick Count (ms)() -> (millisecond timer value=w184:u32)
                      n288 = property on="强度图" class="IntGraph (严格)"("Value"=w177) -> ()  [unwired: 2 in, 2 out]
                      n289 = Subtract(x=w184, y=w183) -> (x-y=w180:u32)
                      n290 = Multiply(x=w180, y=0.001) -> (x*y=→"总用时（s）":dbl)
                      "数组" <- w178
                    }
                  }
                }
              }
            }
          }
        }
        n291 = local read "hDevice out"() -> (w15:i32)
        n292 = dll-call lib="PTH2]abs CUsersH301Desktopart闭环扫描程序采集卡控制INFamd64\nPCI8502_32" fn="PCI8502_ReleaseDeviceAD" label="ReleaseDeviceAD"("hDevice"=w15) -> ("hDevice"=w14:i32)  [unwired: 4 in, 2 out]
        n293 = VISA Close(VISA resource name=w12) -> (error out=→"错误输出":errorcluster)  [unwired: 1 in]
        n294 = dll-call lib="PTH2]abs CUsersH301Desktopart闭环扫描程序采集卡控制INFamd64\nPCI8502_32" fn="PCI8502_ReleaseDevice" label="ReleaseDevice"("hDevice"=w14) -> ()  [unwired: 5 in, 2 out]
        "M_Length" <- w19
      }
    }
  }
  n295 = property on="高级设置" class="Bool"("Visible"=FALSE ("可见")) -> ()  [unwired: 2 in, 2 out]
  n296 = property on="定位模式" class="Bool"("Visible"=FALSE ("可见")) -> ()  [unwired: 2 in, 2 out]
